vi "P_AF.vi"() -> ()   [LabVIEW 2016]
uses:
  <vilib>/Analysis/baseanly.llb/Mean (DBL).vi
  <vilib>/ULx/Create Channel.llb/ULx Create Channel (AI-Voltage-Basic).vi
  <vilib>/ULx/Timing.llb/ULx Timing (Sample Clock).vi
  <vilib>/ULx/Read.llb/ULx Read (Analog 1D Wfm NChan NSamp).vi
  <vilib>/Waveform/WDTOps.llb/WDT Index Channel DBL.vi
  <vilib>/Analysis/NI_AALBase.lvlib
panel:
  out "Flow Rate (SLPS)":dbl
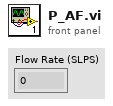
[diagram p1: front panel]
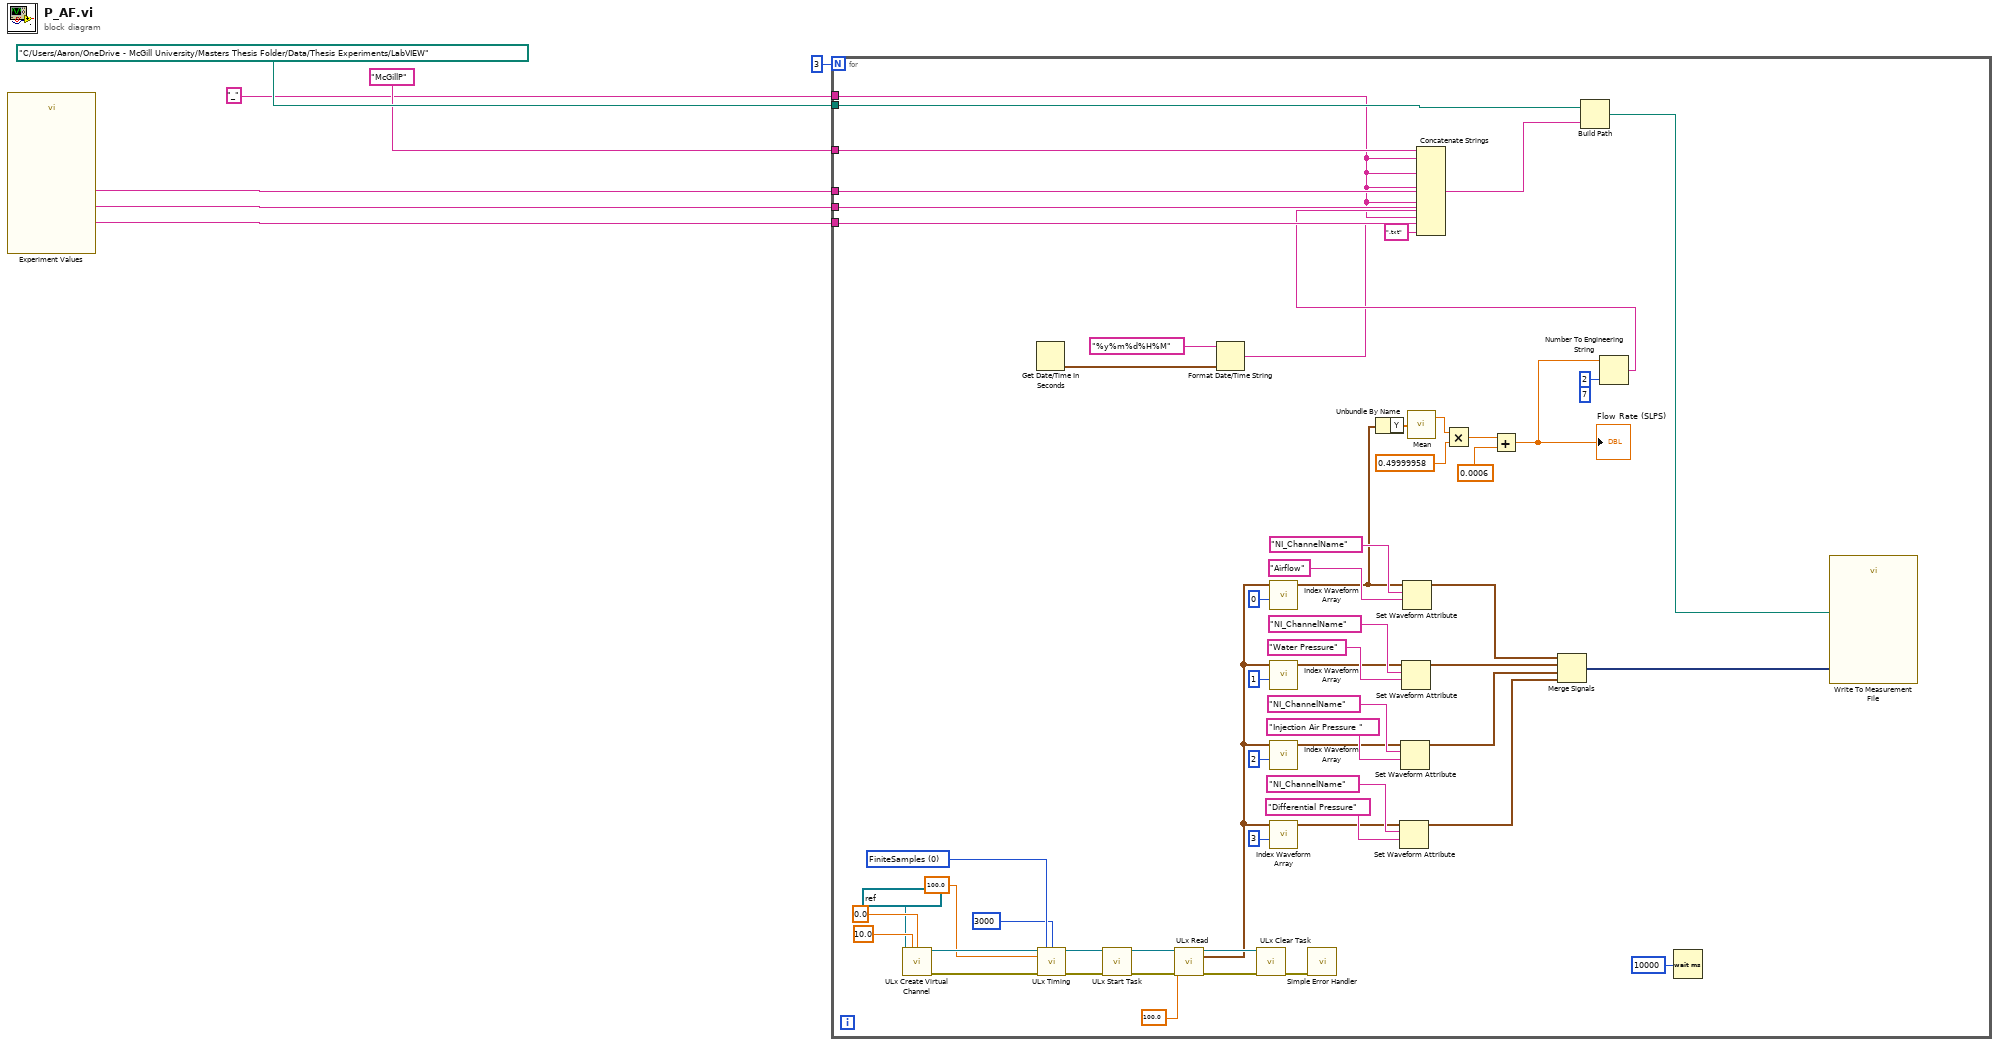
[diagram p0: block diagram]
diagram:
  n1 = call "Experiment Values"() -> ("Water Temperature (C)"=w3:string, "Atmospheric Air Pressure (kPa)"=w4:string, "Water Flowrate (gpm)"=w5:string)  [unwired: 15 in, 2 out]
  n2 = for {
    N: 3 -> [_]
    tunnel: path "C:/Users/Aaron/OneDrive - McGill University/Masters Thesis Folder/Data/Thesis Experiments/LabVIEW" ("Filename") -> [w34]
    tunnel: "McGillP" -> [w29]
    tunnel: w5 -> [w28]
    tunnel: w4 -> [w27]
    tunnel: w3 -> [w26]
    tunnel: "_" -> [w17]
    (unwired) i16 7 ("width (-)")
    w54 = 0 items=["FiniteSamples", "ContinuousSamples"] ("sample mode")
    n3 = call-poly <vilib>:"ULx Create Virtual Channel.vi"("maximum value"=10.0, "minimum value"=0.0, "physical channels"=refnum<k21> "Dev0/Ai7:4") -> ("task out"=w66:refnum<k24>, "error out"=w62:errorcluster)  [unwired: 11 in]
    n4 = Get Date/Time In Seconds() -> (seconds since 1Jan1904=w31:timestamp)
    n5 = call-poly <vilib>:"ULx Timing.vi"("task in"=w66, "sample mode"=w54, "samples per channel"=3000, "rate"=100.0, "error in"=w62) -> ("task out"=w65:refnum<k24>, "error out"=w61:errorcluster)  [unwired: 9 in]
    n6 = call <vilib>:"ULx Start Task.vi"("task in"=w65, "error in"=w61) -> ("task out"=w64:refnum<k24>, "error out"=w60:errorcluster)  [unwired: 12 in]
    n7 = call-poly <vilib>:"ULx Read.vi"("task in"=w64, "timeout"=100.0, "error in"=w60) -> ("task out"=w63:refnum<k24>, "data"=w15:waveform(dbl)[], "error out"=w59:errorcluster)  [unwired: 10 in]
    n8 = Format Date/Time String(time format string (%c)="%y%m%d%H%M", seconds (now)=w31) -> (date/time string=w16:string)  [unwired: 1 in]
    n9 = call <vilib>:"ULx Clear Task.vi"("task in"=w63, "error in"=w59) -> ("error out"=w58:errorcluster)  [unwired: 13 in]
    n10 = call-poly <vilib>:"Index Waveform Array.vi"("index"=0, "waveform array"=w15) -> ("waveform"=w12:waveform(dbl))  [unwired: 8 in, 1 out]
    n11 = call-poly <vilib>:"Index Waveform Array.vi"("index"=1, "waveform array"=w15) -> ("waveform"=w44:waveform(dbl))  [unwired: 8 in, 1 out]
    n12 = call-poly <vilib>:"Index Waveform Array.vi"("index"=2, "waveform array"=w15) -> ("waveform"=w41:waveform(dbl))  [unwired: 8 in, 1 out]
    n13 = call-poly <vilib>:"Index Waveform Array.vi"("index"=3, "waveform array"=w15) -> ("waveform"=w38:waveform(dbl))  [unwired: 8 in, 1 out]
    n14 = call <vilib>:"Simple Error Handler.vi"("error in (no error)"=w58) -> ()  [unwired: 4 in, 5 out]
    n15 = Unbundle By Name(w12) -> ("Y"=w14:dbl[])
    n16 = Set Waveform Attribute(5:"Differential Pressure", 6:"NI_ChannelName" ("name"), 7:w38) -> (3:w36:waveform(dbl))  [unwired: 1 in, 2 out]
    n17 = Set Waveform Attribute(5:"Injection Air Pressure ", 6:"NI_ChannelName" ("name"), 7:w41) -> (3:w37:waveform(dbl))  [unwired: 1 in, 2 out]
    n18 = Set Waveform Attribute(5:"Water Pressure", 6:"NI_ChannelName" ("name"), 7:w44) -> (3:w19:waveform(dbl))  [unwired: 1 in, 2 out]
    n19 = Set Waveform Attribute(5:"Airflow", 6:"NI_ChannelName" ("name"), 7:w12) -> (3:w13:waveform(dbl))  [unwired: 1 in, 2 out]
    n20 = call-poly <vilib>:"Mean.vi"("X"=w14) -> ("mean"=w25:dbl)  [unwired: 1 out]
    n21 = Multiply(x=w25, y=0.49999958) -> (x*y=w23:dbl)
    n22 = Add(x=w23, y=0.0006) -> (x+y=w20:dbl)
    "Flow Rate (SLPS)" <- w20
    n23 = Merge Signals(w13, w19, w37, w36) -> (w35:dynamicdata)
    n24 = Number To Engineering String(2:i16 2 ("precision (6)"), 4:w20) -> (0:w18:string)  [unwired: 2 in]
    n25 = Concatenate Strings(w29, w17, w28, w17, w27, w17, w26, w17, w18, w17, w16, ".txt" ("string")) -> (w32:string)
    n26 = Build Path(base path=w34, name or relative path=w32) -> (appended path=w33:path)
    n27 = Wait (ms)(milliseconds to wait=u32 10000) -> ()  [unwired: 1 out]
    n28 = call "Write To Measurement File"("Signals"=w35, "Filename"=w33) -> ()  [unwired: 15 in, 3 out]
  }
